vi "Initialize Values.vi"(8 "error in (no error)":errorcluster, 11 "AutoZero in":refnum<class "AutoZero.lvclass">) -> (0 "error out":errorcluster, 3 "AutoZero out":refnum<class "AutoZero.lvclass">)   [LabVIEW 2014, in "SeqLoop.lvlib" / "STEP Classes.lvlib" / "AutoZero.lvclass"]
uses:
  AutoZero.lvclass
  AutoZero.lvclass/AutoZero.ctl
  STEP/STEP.lvclass
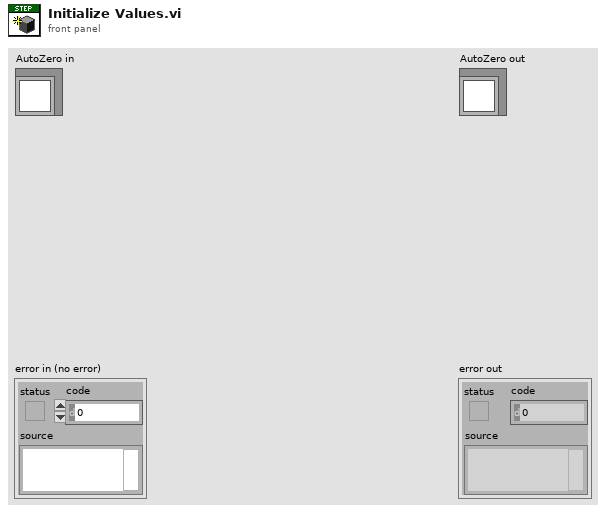
[diagram p1: front panel]
types:
  T1 = cluster{"HWSync 1":bool, "HWSync 2":bool, "HWSync 3":bool, "HWSync 4":bool, "HWSync 5":bool}
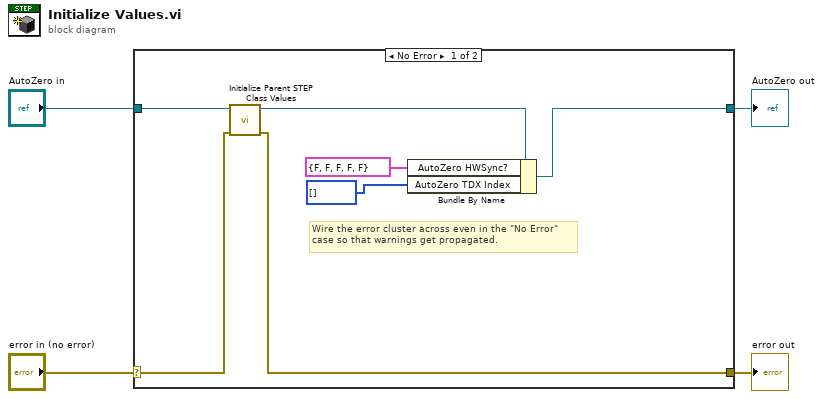
[diagram p0: block diagram]
diagram:
  n1 = case shown="No Error" "error in (no error)" {
    selector: "error in (no error)" -> [w6 w13]
    tunnel: [w5 w13] -> w3
    tunnel: [w9 w12] -> w1
    tunnel: "AutoZero in" -> [w11 w12]
    frame No Error {
      # "Wire the error cluster across even in the \"No Error\"\ncase so that warnings get propagated."
      n2 = call "Initialize Parent STEP Class Values.vi"("error in (no error)"=w6, "STEP in"=w11) -> ("error out"=w5:errorcluster, "STEP out"=w10:refnum<class "AutoZero.lvclass">)  [unwired: 8 in]
      n3 = Bundle By Name(cluster=w10, "AutoZero HWSync?"=T1 {"HWSync 1"=FALSE, "HWSync 2"=FALSE, "HWSync 3"=FALSE, "HWSync 4"=FALSE, "HWSync 5"=FALSE}, "AutoZero TDX Index"=i32[] []) -> (w9:refnum<class "AutoZero.lvclass">)
    }
    frame Error {
    }
  }
  "error out" <- w3
  "AutoZero out" <- w1
